vi "Config Macros.vi"(8 "error in (no error)":errorcluster, 11 "Configuration in":refnum<class "Configuration.lvclass">) -> (0 "error out":errorcluster, 3 "Configuration out":refnum<class "Configuration.lvclass">)   [LabVIEW 2016, in "Hardware.lvlib" / "Motions.lvlib" / "Motions Configuration.lvclass"]
uses:
  <userlib>/Common Components/Hardware/Abstract System/Motions/Motions Config/Motions Configuration.lvclass
  <userlib>/Configuration Dialog Actor/Configuration.lvclass
  <userlib>/TSPopup/TSPopup.Popup Cluster.ctl
  C:/Program Files (x86)/National Instruments/LabVIEW 2016/user.lib/Configuration Dialog Actor/Configuration.lvclass
  C:/Program Files (x86)/National Instruments/LabVIEW 2016/vi.lib/ActorFramework/Actor/Actor.lvclass
  <userlib>/TSPopup/TSPopup.lvclass
  <userlib>/TSPopup/TSPopup.Popup Call Parameters.ctl
  <userlib>/TSPopup/TSPopup.Data Type.ctl
  <userlib>/Common Components/Hardware/Abstract System/Motions/Motions Config/Motions Configuration.lvclass/Motions Configuration.ctl
  <vilib>/ActorFramework/Actor/Actor.lvclass/Actor.ctl
  <userlib>/Common Components/Hardware/Abstract System/Motions/Motions/Motions.lvclass/Motions.ctl
  <userlib>/Common Components/Hardware/Abstract System/Motions/Motions/Motions.lvclass
  <vilib>/ActorFramework/Actor/Actor.lvclass
panel:
  in  "Array of Target Pos":T1(array[cluster])=[{"Label"="X", "Label 2"=FALSE, "Target Pos"=0.0}, {"Label"="Y", "Label 2"=FALSE, "Target Pos"=0.0}, {"Label"="Z", "Label 2"=FALSE, "Target Pos"=0.0}, {"Label"="R1", "Label 2"=FALSE, "Target Pos"=0.0}, {"Label"="R3", "Label 2"=FALSE, "Target Pos"=0.0}]
  in  "Add Item Button":bool
  in  "Remove Item Button":bool
  in  "Save Macro Button":bool
  in  "Popups":T2 {"Boolean" items=["False", "True"]; "Ring" items=["False", "True"]}
  out "Macros List":i32(listbox)
  in  "TA Binding List":i32(listbox)
  in  "Revert":bool
  # "Type Sensitive\nPopup"
  # "Boolean Colors"
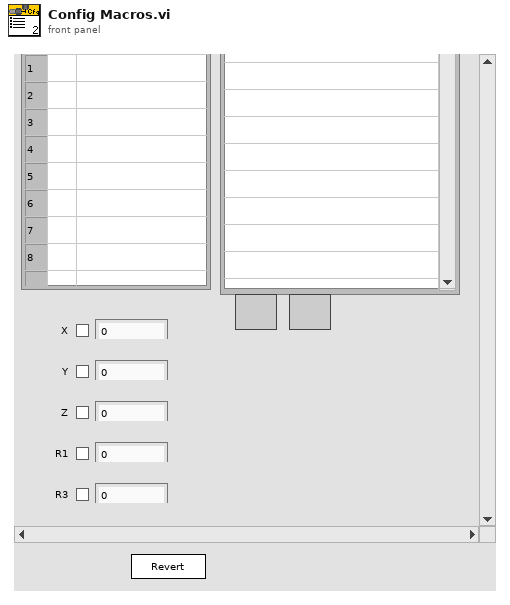
[diagram p1: front panel]
types:
  T1 = cluster{"Label":string, "Label 2":bool, "Target Pos":dbl}[]
  T2 = typedef "TSPopup.lvlib/TSPopup.lvclass/TSPopup.Popup Cluster.ctl" = cluster{"Unknown":bool, "Unknown 2":bool, "String":string, "Integer":i32, "Float":dbl, "Color":u32, "Boolean":u32, "Ring":u32, "Captioned String":cluster{"String":string, "OK":bool, "Cancel":bool}, "Captioned Integer":cluster{"First":i32, "OK":bool, "Cancel":bool}, "Boolean Colors":cluster{"False":cluster{"FG":u32, "BG":u32}, "True":cluster{"FG":u32, "BG":u32}, "T  to  F":cluster{"FG":u32, "BG":u32}, "F  to  T":cluster{"FG":u32, "BG":u32}, "OK":bool, "Cancel":bool}, "2-Int Cluster":cluster{"First":i32, "Second":i32, "OK":bool, "Cancel":bool}, "4-Int Cluster":cluster{"First":i32, "Second":i32, "Third":i32, "Fourth":i32, "OK":bool, "Cancel":bool}, "check":bool}
  T3 = typedef "TSPopup.lvlib/TSPopup.lvclass/TSPopup.Data Type.ctl" = enum16{"Unkown", "NO POPUP", "String", "Integer", "Float", "Color", "Boolean", "Ring", "Captioned String", "Captioned Integer", "Button Color", "2 Int Cluster", "4 Int Cluster", "check"}
  T4 = typedef "TSPopup.lvlib/TSPopup.lvclass/TSPopup.Popup Call Parameters.ctl" = cluster{"Prop Type":T3, "Initial Value":variant, "Caption Strings":string[], "Ring Strings":string[], "Cell Rect":cluster{"left":i16, "top":i16, "right":i16, "bottom":i16}, "Mouse Coords":cluster{"x":i16, "y":i16}, "Call Data":variant}
  T5 = typedef "LVPoint32TypeDef.ctl" = cluster{"Horizontal":i32, "Vertical":i32}
  T6 = typedef "TSPopup.lvlib/TSPopup.lvclass/TSPopup.Grid.Cell Info.ctl" = cluster{"Tag":string, "Row":i32, "Column":i32, "In Symbol?":bool, "In Data?":bool, "Cell String":string, "Ctl Refnum":refnum<vi>, "Prop Type":T3, "Ring Strings":string[]}
  T7 = typedef "Hardware.lvlib/Motions.lvlib/Motions.lvclass/TA Binding Data.ctl" = cluster{"Triggers":cluster{"Triggers for Array AND":cluster{"Index":u8, "State Name":string}[]}[], "Actions":cluster{"Action Name":string, "Action Data":string}[]}
  T8 = typedef "eventvkey.ctl" = enum16{"ASCII", "Enter", "Return", "Shift", "Ctrl", "Alt", "Cmd", "Opt", "Caps", "NumLock", "Clear", "Break", "Up", "Down", "Left", "Right", "Insert", "Delete", "Home", "End", "PageUp", "PageDown", "Escape", "Help", "Pause", "ScrollLock", "F1", "F2", "F3", "F4", "F5", "F6", "F7", "F8", "F9", "F10", "F11", "F12", "F13", "F14", "F15", "F16", "F17", "F18", "F19", "F20", "F21", "F22", "F23", "F24", "Play", "VolumeUp", "VolumeDown", "Mute", "Two Byte Char"}
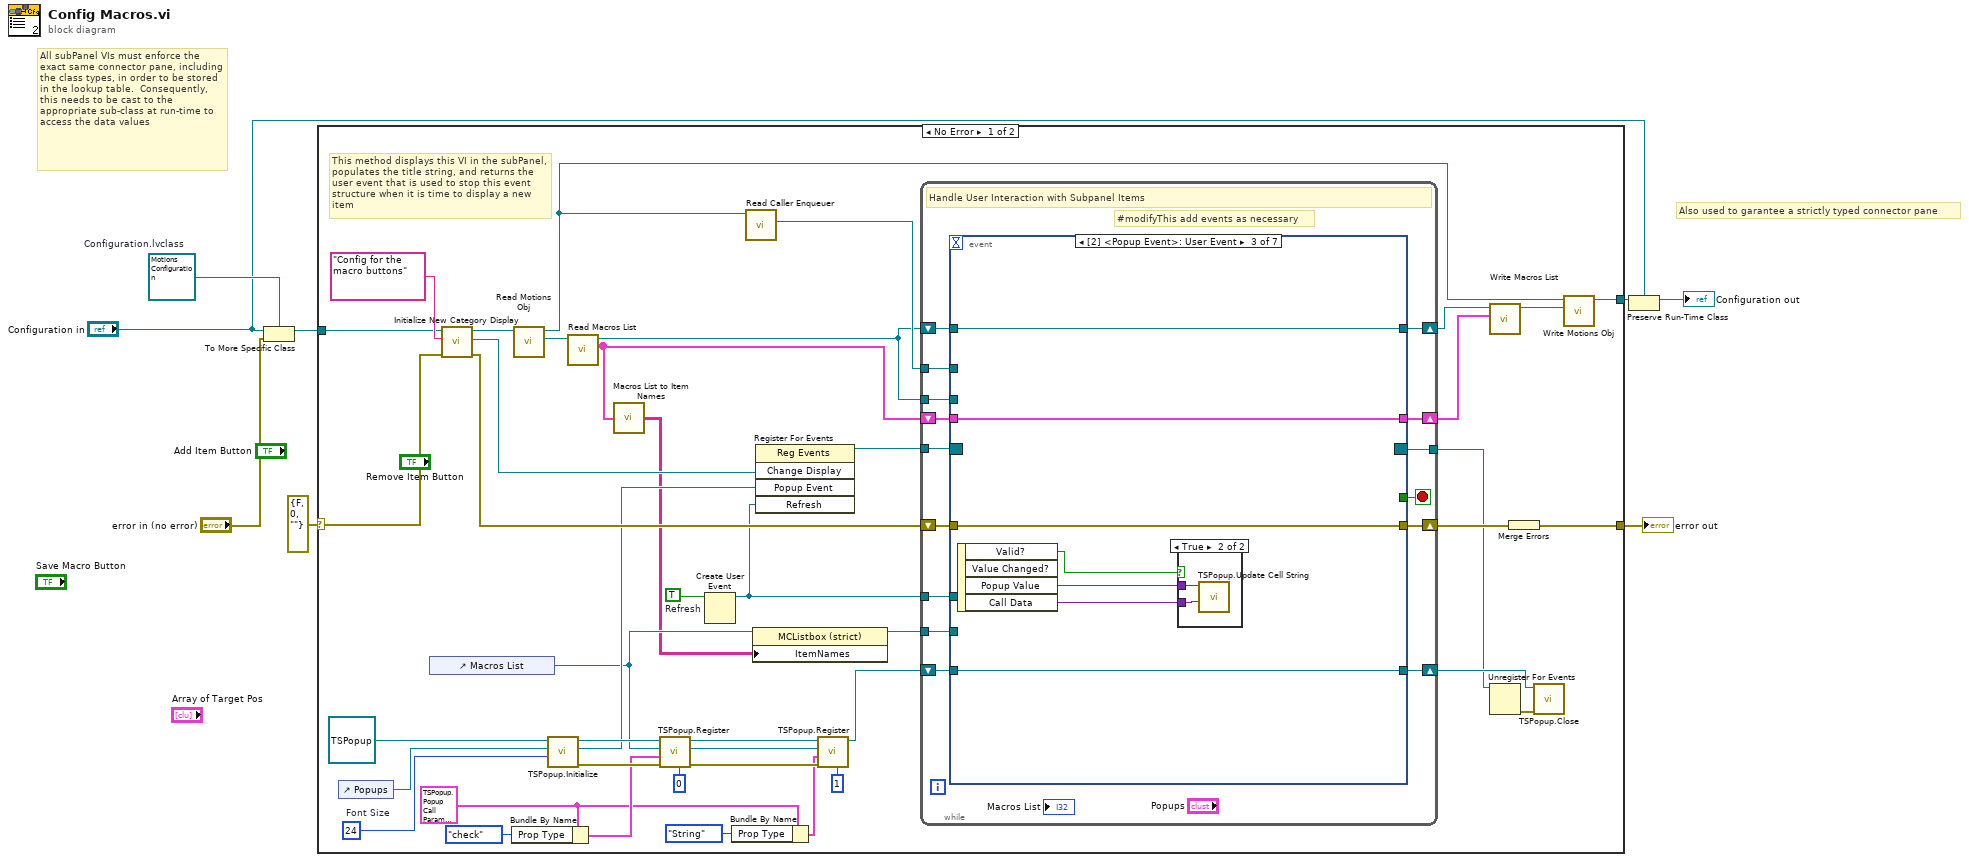
[diagram p0: block diagram]
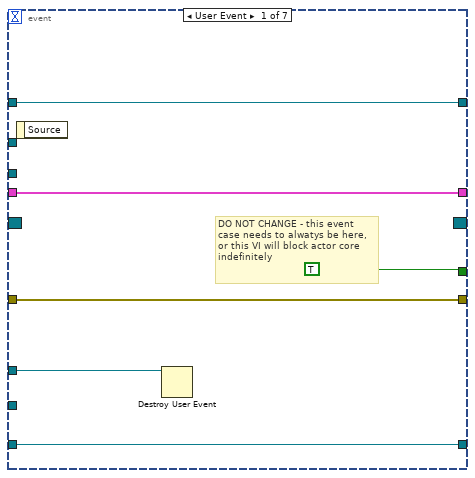
[diagram p2: hidden frame]
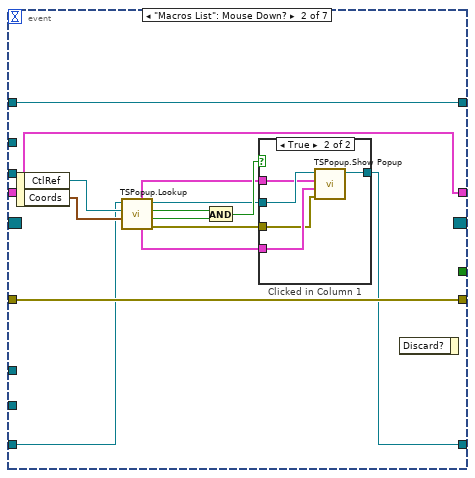
[diagram p3: hidden frame]
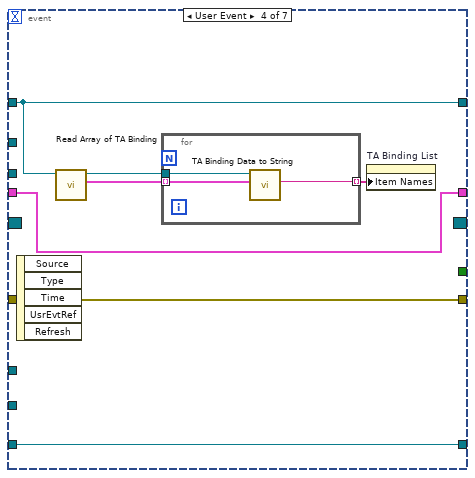
[diagram p6: hidden frame]
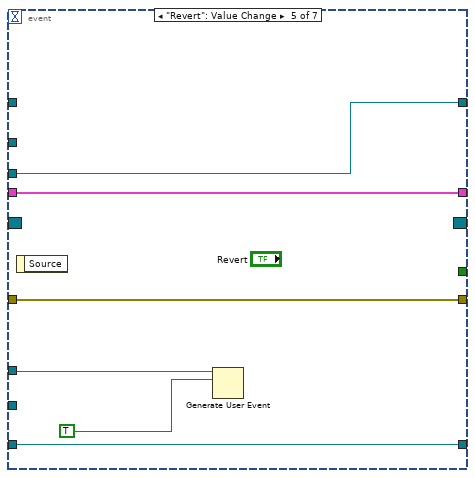
[diagram p7: hidden frame]
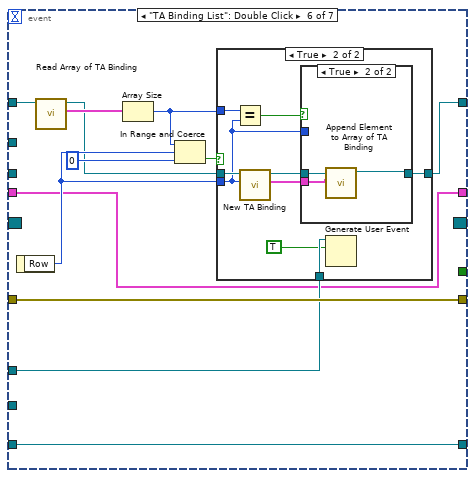
[diagram p8: hidden frame]
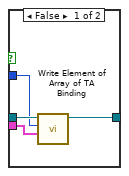
[diagram p10: hidden frame]
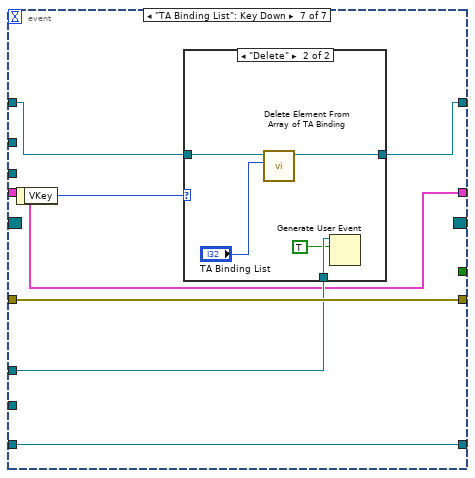
[diagram p11: hidden frame]
diagram:
  w5 = refnum<class "Motions Configuration.lvclass"> refnum  # Configuration.lvclass
  # "Also used to garantee a strictly typed connector pane"
  # "All subPanel VIs must enforce the exact same connector pane, including the class types, in order to be stored in the lookup table.  Consequently, this needs to be cast to the appropriate sub-class at run-time to access the data values"
  n1 = To More Specific Class(target class=w5, reference="Configuration in", error in="error in (no error)") -> (specific class reference=w6:refnum<class "Motions Configuration.lvclass">)  [unwired: 1 out]
  n2 = case shown="No Error" errorcluster {"status"=FALSE, "code"=0, "source"=""} ("error IO") {
    selector: errorcluster {"status"=FALSE, "code"=0, "source"=""} ("error IO") -> [w50 w160]
    tunnel: w6 -> [w43 w161]
    tunnel: [w37 w161] -> w8
    tunnel: [w51 w160] -> w7
    frame No Error {
      w21 = T4 {"Prop Type"=enum."Unkown", "Initial Value"=variant, "Caption Strings"=[], "Ring Strings"=[], "Cell Rect"={"left"=0, "top"=0, "right"=0, "bottom"=0}, "Mouse Coords"={"x"=0, "y"=0}, "Call Data"=variant} ("Show Popup (type only)")
      w32 = u32 24  # Font Size
      w42 = TRUE  # Refresh
      # "This method displays this VI in the subPanel, populates the title string, and returns the user event that is used to stop this event structure when it is time to display a new item"
      n3 = control-ref of="Popups"() -> (w35:refnum<vi>)
      n4 = control-ref of="Macros List"() -> (w29:refnum<vi>)
      n5 = call <userlib>:"Initialize New Category Display.vi"("error in (no error)"=w50, "Name to Display"="Config for the macro buttons", "Configuration in"=w43) -> ("error out"=w45:errorcluster, "Change Display"=w48:refnum<user-event>, "Configuration Out"=w39:refnum<class "Motions Configuration.lvclass">)  [unwired: 6 in]
      n6 = Bundle By Name(cluster=w21, "Prop Type"=TSPopup.Data_Type."check") -> (w26:T4)
      n7 = call <userlib>:"Read Motions Obj.vi"("Motions Configuration in"=w39) -> ("Hardware.lvlib:Motions.lvlib:Motions.lvclass"=w40:refnum<class "Motions.lvclass">, "Motions Configuration out"=w38:refnum<class "Motions Configuration.lvclass">)  [unwired: 8 in, 1 out]
      n8 = call <userlib>:"TSPopup.Initialize.vi"("Font Size"=w32, "Popup Cluster Ref"=w35, "TSPopup in"=refnum<class "TSPopup.lvclass"> refnum ("TSPopup.lvclass")) -> ("error out"=w34:errorcluster, "Popup Event"=w30:refnum<user-event>, "TSPopup out"=w33:refnum<class "TSPopup.lvclass">)  [unwired: 6 in]
      n9 = call <userlib>:"Read Macros List.vi"("Motions in"=w40) -> ("Macros List"=w9:cluster{"enabled?":bool, "macro name":string}[], "Motions out"=w13:refnum<class "Motions.lvclass">)  [unwired: 9 in]
      n10 = call <userlib>:"Macros List to Item Names.vi"("Macros List"=w9) -> ("Item Names"=w12:string[][])
      n11 = call <userlib>:"TSPopup.Register.vi"("Col (unwired = all columns)"=0, "error in (no error)"=w34, "Parameters"=w26, "Ctl Refnum"=w29, "TSPopup in"=w33) -> ("error out"=w22:errorcluster, "dup ref out"=w18:refnum<vi>, "TSPopup out"=w23:refnum<class "TSPopup.lvclass">)  [unwired: 4 in]
      n12 = Create User Event(user event datatype=w42) -> (user event=w41:refnum<user-event>)  [unwired: 1 in, 1 out]
      n13 = Bundle By Name(cluster=w21, "Prop Type"=TSPopup.Data_Type."String") -> (w19:T4)
      n14 = call <vilib>:"Read Caller Enqueuer.vi"("Actor"=w38) -> ("Caller Enqueuer"=w44:refnum<class "Message Enqueuer.lvclass">)  [unwired: 10 in]
      n15 = property class="MCListbox (strict)"(reference=w29, "ItemNames"=w12) -> (reference out=w28:refnum<vi>)  [unwired: 1 in, 1 out]
      n16 = register-events(w48, w30, w41) -> (reference out=w47:refnum<event-registration>)  [unwired: 2 in, 1 out]
      n17 = call <userlib>:"TSPopup.Register.vi"("Col (unwired = all columns)"=1, "error in (no error)"=w22, "Parameters"=w19, "Ctl Refnum"=w18, "TSPopup in"=w23) -> ("TSPopup out"=w17:refnum<class "TSPopup.lvclass">)  [unwired: 4 in, 2 out]
      n18 = while {
        tunnel: w47 -> [w65]
        shift-right: [w64] -> w46
        shift-left: w45 -> [w63]
        tunnel: w44 -> [w62]
        tunnel: w13 -> [w61]
        tunnel: w41 -> [w60]
        shift-right: [w58] -> w36
        shift-left: w13 -> [w59]
        tunnel: w28 -> [w57]
        shift-right: [w54] -> w15
        shift-left: w17 -> [w56]
        tunnel: [w55] -> w14
        shift-right: [w52] -> w10
        shift-left: w9 -> [w53]
        stop <- w66 stop-if-true
        # "#modifyThis add events as necessary"
        # "Handle User Interaction with Subpanel Items"
        n19 = event shown="[2] <Popup Event>: User Event" {
          selector: w65 -> [_ _ _ _ _ _ _]
          dyn-events: [_ _ _ _ _ _ _] -> w55
          timeout: _ -> [_ _ _ _ _ _ _]
          tunnel: [TRUE _ _ _ _ _ _] -> w66
          tunnel: [w72 w86 w99 w108 w117 w129 w153] -> w64
          tunnel: w63 -> [w72 w86 w99 w108 w117 w129 w153]
          tunnel: w62 -> [_ _ _ _ _ _ _]
          tunnel: w61 -> [_ _ _ _ w114 _ _]
          tunnel: w60 -> [w70 _ _ _ w116 w124 w151]
          tunnel: w59 -> [w69 w85 w98 w106 _ w122 w150]
          tunnel: [w69 w85 w98 w106 w114 w121 w149] -> w58
          tunnel: w57 -> [_ _ _ _ _ _ _]
          tunnel: w56 -> [w68 w75 w97 w103 w113 w119 w148]
          tunnel: [w68 w74 w97 w103 w113 w119 w148] -> w54
          tunnel: w53 -> [w67 w73 w93 w102 w112 w118 w147]
          tunnel: [w67 w73 w93 w102 w112 w118 w147] -> w52
          event User Event {
            # "DO NOT CHANGE - this event case needs to alwatys be here, or this VI will block actor core indefinitely"
            n20 = event-data() -> ()  [unwired: 1 in, 1 out]
            n21 = Destroy User Event(user event=w70) -> ()  [unwired: 1 in, 1 out]
          }
          event "Macros List": Mouse Down? {
            n22 = event-data() -> ("CtlRef"=w77:refnum<vi>, "Coords"=w76:T5)  [unwired: 1 in]
            n23 = call <userlib>:"TSPopup.Lookup.vi"("Point"=w76, "Ctl Refnum"=w77, "TSPopup in"=w75) -> ("error out"=w80:errorcluster, "In Bounds?"=w81:bool, "Found"=w82:bool, "TSPopup out"=w78:refnum<class "TSPopup.lvclass">, "Cell Info (Call data)"=w79:T6, "Popup Parameters"=w83:T4)  [unwired: 3 in]
            n24 = And(x=w82, y=w81) -> (x .and. y?=w84:bool)
            n25 = case "Clicked in Column 1" shown="True" w84 {
              tunnel: w83 -> [_ w88]
              tunnel: w79 -> [_ w90]
              tunnel: w80 -> [_ w89]
              tunnel: w78 -> [w87 w92]
              tunnel: [w87 w91] -> w74
              frame False {
              }
              frame True {
                n26 = call <userlib>:"TSPopup.Show Popup.vi"("error in (no error)"=w89, "Call Data (ignore if empty)"=w90, "Popup Parameters"=w88, "TSPopup in"=w92) -> ("TSPopup out"=w91:refnum<class "TSPopup.lvclass">)  [unwired: 6 in, 1 out]
              }
            }
            n27 = event-data() -> ()  [unwired: 2 in, 1 out]
          }
          event User Event {
            n28 = event-data() -> ("Valid?"=w96:bool, "Popup Value"=w94:variant, "Call Data"=w95:variant)  [unwired: 1 in, 1 out]
            n29 = case shown="True" w96 {
              tunnel: w94 -> [_ w100]
              tunnel: w95 -> [_ w101]
              frame False {
              }
              frame True {
                n30 = call <userlib>:"TSPopup.Update Cell String.vi"("Call Data (must be Cell Info cluster)"=w101, "Popup Value"=w100) -> ()  [unwired: 9 in, 1 out]
              }
            }
          }
          event User Event {
            n31 = event-data() -> ()  [unwired: 1 in, 5 out]
            n32 = call <userlib>:"Read Array of TA Binding.vi"("Motions in"=w106) -> ("Array of TA Binding"=w104:T7[], "Motions out"=w105:refnum<class "Motions.lvclass">)  [unwired: 9 in]
            n33 = for {
              tunnel: w104 -> [w111] mode=indexing
              tunnel: [w110] -> w107 mode=indexing
              tunnel: w105 -> [w109]
              n34 = call <userlib>:"TA Binding Data to String.vi"("TA Binding Data"=w111, "Motions in"=w109) -> ("String"=w110:string)  [unwired: 7 in, 2 out]
            }
            n35 = property on="TA Binding List" class="LstBox (strict)"("Item Names"=w107) -> ()  [unwired: 2 in, 2 out]
          }
          event "Revert": Value Change {
            n36 = event-data() -> ()  [unwired: 1 in, 1 out]
            n37 = Generate User Event(user event=w116, event data cluster=TRUE) -> ()  [unwired: 2 in, 2 out]
          }
          event "TA Binding List": Double Click {
            n38 = event-data() -> ("Row"=w128:i32)  [unwired: 1 in]
            n39 = call <userlib>:"Read Array of TA Binding.vi"("Motions in"=w122) -> ("Array of TA Binding"=w123:T7[], "Motions out"=w120:refnum<class "Motions.lvclass">)  [unwired: 9 in]
            n40 = Array Size(array=w123) -> (size(s)=w125:i32)
            n41 = In Range and Coerce(upper limit=w125, x=w128, lower limit=0) -> (In Range?=w126:bool)  [unwired: 1 out]
            n42 = case shown="True" w126 {
              tunnel: w120 -> [w130 w139]
              tunnel: w128 -> [_ w135]
              tunnel: w125 -> [_ w138]
              tunnel: w124 -> [_ w134]
              tunnel: [w130 w131] -> w121
              frame False {
              }
              frame True {
                n43 = Equal?(x=w138, y=w135) -> (x = y?=w137:bool)
                n44 = call <userlib>:"New TA Binding.vi"("Index (out of array range means creating new)"=w135, "Motions in"=w139) -> ("New TA Binding out"=w136:T7, "Motions out"=w132:refnum<class "Motions.lvclass">)  [unwired: 7 in, 1 out]
                n45 = case shown="True" w137 {
                  tunnel: w136 -> [w142 w145]
                  tunnel: w135 -> [w141 _]
                  tunnel: w132 -> [w143 w146]
                  tunnel: [w140 w144] -> w131
                  frame False {
                    n46 = call <userlib>:"Write Element of Array of TA Binding.vi"("Cluster"=w142, "index"=w141, "Motions in"=w143) -> ("Motions out"=w140:refnum<class "Motions.lvclass">)  [unwired: 8 in]
                  }
                  frame True {
                    n47 = call <userlib>:"Append Element to Array of TA Binding.vi"("Cluster"=w145, "Motions in"=w146) -> ("Motions out"=w144:refnum<class "Motions.lvclass">)  [unwired: 9 in]
                  }
                }
                n48 = Generate User Event(user event=w134, event data cluster=TRUE) -> ()  [unwired: 2 in, 2 out]
              }
            }
          }
          event "TA Binding List": Key Down {
            n49 = event-data() -> ("VKey"=w152:T8)  [unwired: 1 in]
            n50 = case shown="\"Delete\"" w152 {
              tunnel: w151 -> [_ w159]
              tunnel: w150 -> [w154 w157]
              tunnel: [w154 w156] -> w149
              frame Default {
              }
              frame "Delete" {
                n51 = call <userlib>:"Delete Element From Array of TA Binding.vi"("index"="TA Binding List", "Motions in"=w157) -> ("Motions out"=w156:refnum<class "Motions.lvclass">)  [unwired: 9 in]
                n52 = Generate User Event(user event=w159, event data cluster=TRUE) -> ()  [unwired: 2 in, 2 out]
              }
            }
          }
        }
      }
      n53 = call <userlib>:"Write Macros List.vi"("Macros List"=w10, "Motions in"=w36) -> ("Motions out"=w11:refnum<class "Motions.lvclass">)  [unwired: 9 in]
      n54 = Unregister For Events(event registration refnum=w14) -> (error out=w16:errorcluster)  [unwired: 1 in]
      n55 = Merge Errors(w46) -> (w51:errorcluster)
      n56 = call <userlib>:"TSPopup.Close.vi"("error in (no error)"=w16, "TSPopup in"=w15) -> ()  [unwired: 8 in, 2 out]
      n57 = call <userlib>:"Write Motions Obj.vi"("Hardware.lvlib:Motions.lvlib:Motions.lvclass"=w11, "Motions Configuration in"=w38) -> ("Motions Configuration out"=w37:refnum<class "Motions Configuration.lvclass">)  [unwired: 8 in, 1 out]
    }
    frame Error {
    }
  }
  "error out" <- w7
  n58 = Preserve Run-Time Class(object in=w8, 2:"Configuration in") -> (object out=→"Configuration out":refnum<class "Configuration.lvclass">)  [unwired: 1 in, 1 out]
